vi "sv_Subtract Delta Phase.vi"(5 "phase in [deg]":dbl, 7 "frequency [Hz]":dbl, 9 "dt [s]":dbl) -> (8 "phase out [deg]":dbl)   [LabVIEW 2017, in "SoundVib_Generation.lvlib"]
uses:
  <vilib>/addons/_NISVFA/_Generation/SoundVib_Generation.lvlib
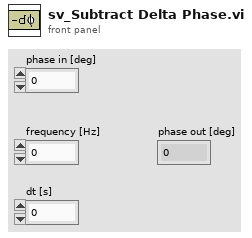
[diagram p1: front panel]
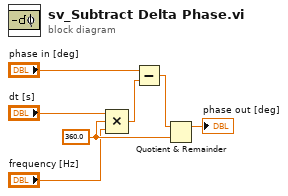
[diagram p0: block diagram]
diagram:
  w5 = 360.0 ("value")
  n1 = Compound Arithmetic op=MULTIPLY("dt [s]", w5, "frequency [Hz]") -> (w7:dbl)
  n2 = Subtract(x="phase in [deg]", y=w7) -> (x-y=w6:dbl)
  n3 = Quotient & Remainder(x=w6, y=w5) -> (x-y*floor(x/y)=→"phase out [deg]":dbl)  [unwired: 1 out]
